vi "Init_library.vi"(8 "error in":errorcluster) -> (0 "error out":errorcluster)   [LabVIEW 2019, in "PICam.lvlib"]
doc: "Picam_InitializeLibrary() initializes the library and prepares it for use."
uses:
  PICam.lvlib
  Picam64.dll   
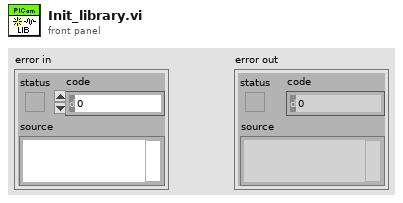
[diagram p1: front panel]
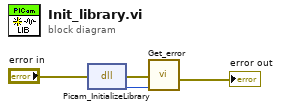
[diagram p0: block diagram]
diagram:
  n1 = dll-call lib="Picam32.dll" fn="Picam_InitializeLibrary"(error in="error in") -> (error out=w3:errorcluster, "return type"=w2:i32)  [unwired: 2 in, 1 out]
  n2 = call "Get_error.vi"("PICam_Error"=w2, "error in (no error)"=w3) -> ("error out"=→"error out":errorcluster)  [unwired: 9 in]
